vi "Quote_path.vi"(1 "File path in":path) -> (0 "result string":string)   [LabVIEW 2025]
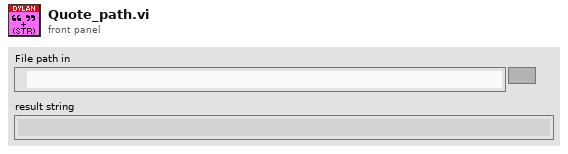
[diagram p1: front panel]
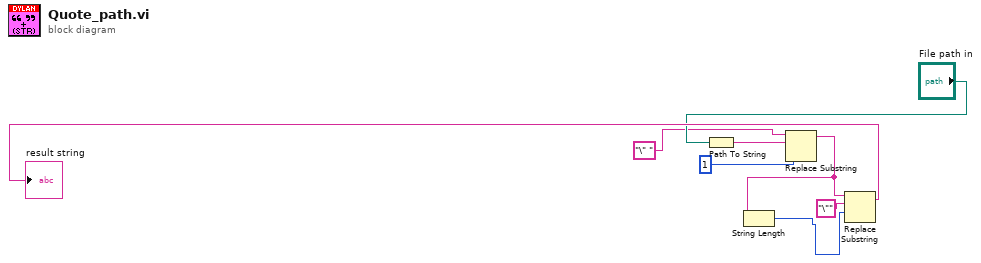
[diagram p0: block diagram]
diagram:
  n1 = Path To String(path="File path in") -> (string=w3:string)
  n2 = Replace Substring(3:1 ("offset (0)"), 4:w3, 5:"\" " ("substring (\"\")")) -> (1:w2:string)  [unwired: 1 in, 1 out]
  n3 = String Length(string=w2) -> (length=w1:i32)
  n4 = Replace Substring(3:w1, 4:"\"" ("substring (\"\")"), 5:w2) -> (1:→"result string":string)  [unwired: 1 in, 1 out]
